vi "Set AIM Hardware Parameters.vi"(8 "error in":errorcluster, 10 "aim hardware parameters":T1={"initialization method"=enum."PXI Slot Number", "card number"=0, "pxi slot number"=2, "biu number"=0, "bus selection"=enum."Both", "coupling mode"=enum."Isolated Onboard Termination", "timing mode"=enum."Disabled (Relative Timestamps)"}, 11 "custom device":T6=18446744073709551615 format="%.0x") -> (0 "error out":errorcluster, 3 "custom device out":T6 format="%.0x")   [LabVIEW 2020, in "AIM MIL-STD-1553 Scripting.lvlib"]
doc: "Configures <b>aim hardware parameters</b> such as PXI Slot Number and BIU Number in the system definition for the specified <b>custom device</b>."
uses:
  AIM MIL-STD-1553 Scripting.lvlib
  <vilib>/NI VeriStand/Custom Device API/Custom Device Item Ref.ctl
  Shared/AIM Hardware Parameters.ctl
  Shared/Initialization Method.ctl
  Shared/Bus Selection.ctl
  Shared/Coupling Mode.ctl
  Constants.vi
  <vilib>/NI VeriStand/Custom Device API/Set Item Property (U16).vi
  <vilib>/NI VeriStand/Custom Device API/Set Item Property (I32).vi
  <vilib>/NI VeriStand/Custom Device API/Custom Device API.lvlib
  Shared/Timing Mode.ctl
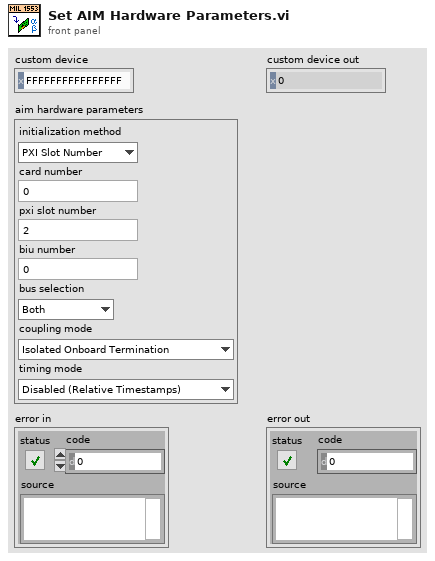
[diagram p1: front panel]
types:
  T1 = typedef "AIM Hardware Parameters.ctl" = cluster{"initialization method":T2, "card number":i32, "pxi slot number":i32, "biu number":i32, "bus selection":T3, "coupling mode":T4, "timing mode":T5}
  T2 = typedef "Initialization Method.ctl" = enum16{"PXI Slot Number", "Card Number"}
  T3 = typedef "Bus Selection.ctl" = enum16{"Both", "Primary", "Secondary"}
  T4 = typedef "Coupling Mode.ctl" = enum16{"Isolated Onboard Termination", "Transformer Coupled", "Direct Coupled", "External with Onboard Termination", "Onboard Digital Wrap-around"}
  T5 = typedef "Timing Mode.ctl" = enum16{"Disabled (Relative Timestamps)", "IRIG (Internal Source)", "IRIG (External Source)", ""}
  T6 = typedef "Custom Device API.lvlib/Custom Device Item Ref.ctl" = u64
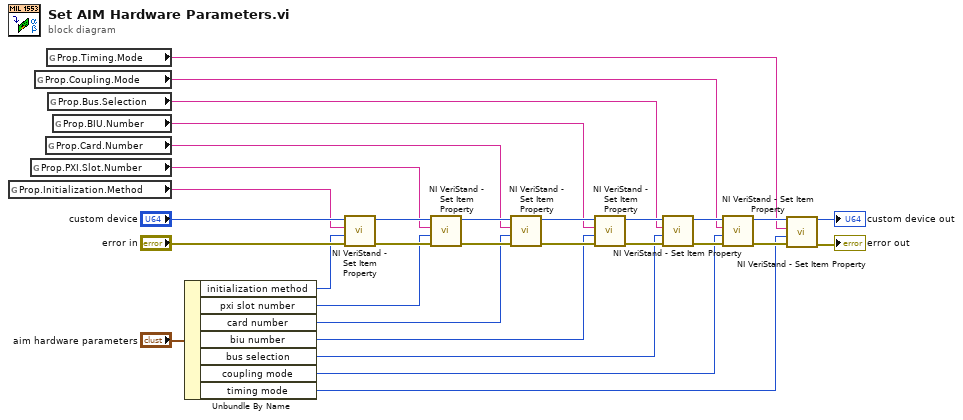
[diagram p0: block diagram]
diagram:
  n1 = global read "Constants.vi" "Prop.Initialization.Method"() -> (w19:string)
  n2 = global read "Constants.vi" "Prop.PXI.Slot.Number"() -> (w18:string)
  n3 = global read "Constants.vi" "Prop.Coupling.Mode"() -> (w9:string)
  n4 = global read "Constants.vi" "Prop.Card.Number"() -> (w17:string)
  n5 = global read "Constants.vi" "Prop.Timing.Mode"() -> (w2:string)
  n6 = global read "Constants.vi" "Prop.Bus.Selection"() -> (w10:string)
  n7 = global read "Constants.vi" "Prop.BIU.Number"() -> (w16:string)
  n8 = Unbundle By Name("aim hardware parameters") -> ("initialization method"=w23:T2, "pxi slot number"=w22:i32, "card number"=w21:i32, "biu number"=w20:i32, "bus selection"=w7:T3, "coupling mode"=w8:T4, "timing mode"=w1:T5)
  n9 = call-poly <vilib>:"NI VeriStand - Set Item Property.vi"("error in (no error)"="error in", "Value"=w23, "Property Name"=w19, "Item Ref in"="custom device") -> ("error out"=w25:errorcluster, "Item Ref out"=w24:T6)  [unwired: 5 in, 1 out]
  n10 = call-poly <vilib>:"NI VeriStand - Set Item Property.vi"("error in (no error)"=w25, "Value"=w22, "Property Name"=w18, "Item Ref in"=w24) -> ("error out"=w30:errorcluster, "Item Ref out"=w31:T6)  [unwired: 5 in, 1 out]
  n11 = call-poly <vilib>:"NI VeriStand - Set Item Property.vi"("error in (no error)"=w30, "Value"=w21, "Property Name"=w17, "Item Ref in"=w31) -> ("error out"=w28:errorcluster, "Item Ref out"=w29:T6)  [unwired: 5 in, 1 out]
  n12 = call-poly <vilib>:"NI VeriStand - Set Item Property.vi"("error in (no error)"=w28, "Value"=w20, "Property Name"=w16, "Item Ref in"=w29) -> ("error out"=w12:errorcluster, "Item Ref out"=w11:T6)  [unwired: 5 in, 1 out]
  n13 = call-poly <vilib>:"NI VeriStand - Set Item Property.vi"("error in (no error)"=w12, "Value"=w7, "Property Name"=w10, "Item Ref in"=w11) -> ("error out"=w14:errorcluster, "Item Ref out"=w13:T6)  [unwired: 5 in, 1 out]
  n14 = call-poly <vilib>:"NI VeriStand - Set Item Property.vi"("error in (no error)"=w14, "Value"=w8, "Property Name"=w9, "Item Ref in"=w13) -> ("error out"=w6:errorcluster, "Item Ref out"=w4:T6)  [unwired: 5 in, 1 out]
  n15 = call-poly <vilib>:"NI VeriStand - Set Item Property.vi"("error in (no error)"=w6, "Value"=w1, "Property Name"=w2, "Item Ref in"=w4) -> ("error out"=→"error out":errorcluster, "Item Ref out"=→"custom device out":T6)  [unwired: 5 in, 1 out]
